vi "Panel.vi"(11 "Element A in":refnum<class "Element B.lvclass">) -> ()   [LabVIEW 2020, in "Array Example.lvlib" / "Element B.lvclass"]
uses:
  Element B.lvclass
  C:/dev/IlluminatedG/lv-oopanel/Examples/Array/Element Base/Element Base.lvclass
  C:/dev/IlluminatedG/lv-oopanel/OOPanel/Panel/Panel.lvclass
  OOPanel/OOPanel.lvlib
  OOPanel/Panel/Panel.lvclass
  Element Base/Element Base.lvclass
panel:
  in  "Numeric":dbl
  out "ID":i32
  out "i":i32
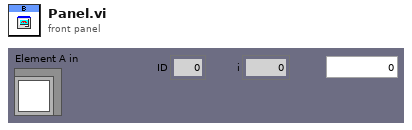
[diagram p1: front panel]
types:
  T1 = typedef "OOPanel.lvlib/Panel.lvclass/Visibility State.ctl" = enum16{"Idle", "Closed", "Hidden", "Visible", "Subpanel"}
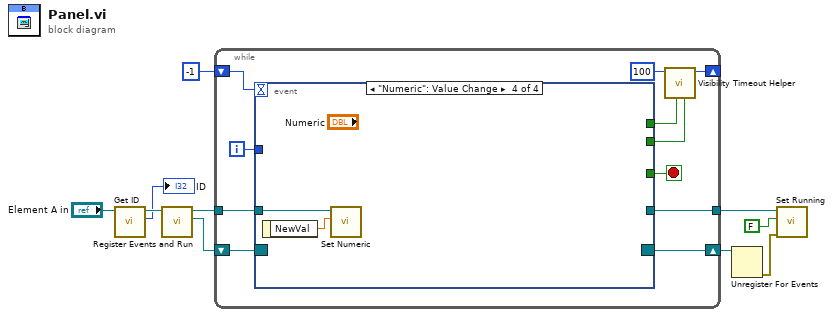
[diagram p0: block diagram]
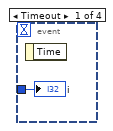
[diagram p2: hidden frame]
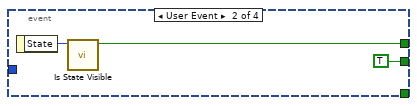
[diagram p3: hidden frame]
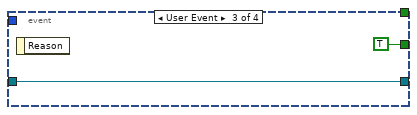
[diagram p4: hidden frame]
diagram:
  n1 = call "Get ID.vi"("Element Base in"="Element A in") -> ("ID"=→"ID":i32, "Element Base out"=w6:refnum<class "Element B.lvclass">)  [unwired: 8 in, 1 out]
  n2 = call "Register Events and Run.vi"("Panel in"=w6) -> ("Panel Event Reg"=w10:refnum<event-registration>, "Panel out"=w9:refnum<class "Element B.lvclass">)  [unwired: 8 in, 1 out]
  n3 = while {
    shift-right: [w16] -> w2
    shift-left: w10 -> [w21]
    tunnel: w9 -> [w12]
    shift-right: [w19] -> _
    shift-left: -1 -> [w20]
    tunnel: [w11] -> w4
    i -> [w17]
    stop <- w13 stop-if-true
    n4 = event shown="[3] \"Numeric\": Value Change" {
      selector: w21 -> [_ _ _ _]
      dyn-events: [_ _ _ _] -> w16
      timeout: w20 -> [_ _ _ _]
      tunnel: w17 -> [w22 _ _ _]
      tunnel: [_ w24 _ _] -> w15
      tunnel: [_ TRUE _ _] -> w14
      tunnel: [_ _ TRUE _] -> w13
      tunnel: w12 -> [_ _ w26 w29]
      tunnel: [_ _ w26 _] -> w11
      event Timeout {
        n5 = event-data() -> ()  [unwired: 1 in, 1 out]
        "i" <- w22
      }
      event User Event {
        n6 = event-data() -> ("State"=w25:T1)  [unwired: 1 in]
        n7 = call "Is State Visible.vi"("Visibility"=w25) -> ("Visible"=w24:bool)  [unwired: 10 in]
      }
      event User Event {
        n8 = event-data() -> ()  [unwired: 1 in, 1 out]
      }
      event "Numeric": Value Change {
        n9 = event-data() -> ("NewVal"=w28:dbl)  [unwired: 1 in]
        n10 = call "Set Numeric.vi"("Numeric"=w28, "Element A in"=w29) -> ()  [unwired: 8 in, 2 out]
      }
    }
    n11 = call "Visibility Timeout Helper.vi"("Update?"=w14, "Use Timeout?"=w15, "Visible Timeout mS"=100) -> ("Timeout"=w19:i32)  [unwired: 8 in]
  }
  n12 = Unregister For Events(event registration refnum=w2) -> (error out=w1:errorcluster)  [unwired: 1 in]
  n13 = call "Set Running.vi"("error in (no error)"=w1, "Running"=FALSE, "Panel in"=w4) -> ()  [unwired: 7 in, 2 out]
